vi "FitsFormatHeaderText.vi"(8 "error in (no error)":errorcluster, 9 "Keyword Value":string, 10 "Keyword Name":string, 11 "CFitsIO in":refnum<class "CFitsIO.lvclass">) -> (0 "error out":errorcluster, 2 "result string":string, 3 "CFitsIO out":refnum<class "CFitsIO.lvclass">)   [LabVIEW 2016, in "CFitsIO.lvclass"]
uses:
  CFitsIO.lvclass
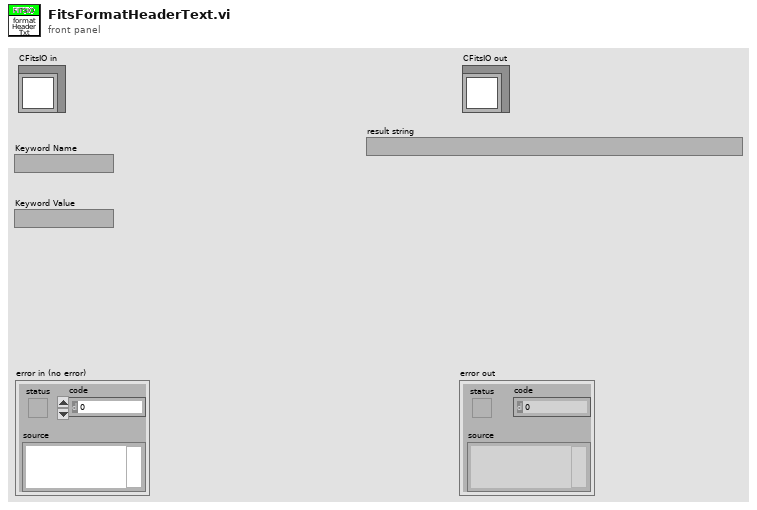
[diagram p1: front panel]
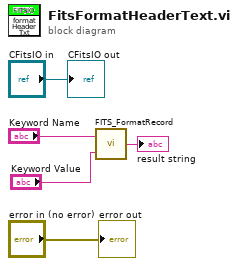
[diagram p0: block diagram]
diagram:
  n1 = call "FITS_FormatRecord.vi"("Keyword Value"="Keyword Value", "Keyword Name"="Keyword Name") -> ("result string"=→"result string":string)
  "error out" <- "error in (no error)"
  "CFitsIO out" <- "CFitsIO in"
